vi "Broadcast Origin.vi"(8 "error in (no error)":errorcluster, 11 "Yaml Model in":refnum<class "Yaml Model.lvclass">) -> (0 "error out":errorcluster, 3 "Yaml Model out":refnum<class "Yaml Model.lvclass">)   [LabVIEW 2020, in "Yaml Model.lvlib" / "Yaml Model.lvclass"]
uses:
  Yaml Model.lvclass
  Yaml Model Messages/Abstract Origin Msg/Abstract Origin Msg.lvclass
  C:/Program Files/National Instruments/LabVIEW 2020/vi.lib/ActorFrameworkObserver/Data Message/Data Message.lvclass
  Yaml Model.lvclass/Yaml Model.ctl
  <vilib>/ActorFrameworkObserver/Actor Register/Actor Register.lvclass
panel:
  # "NOTICE -- YOU MUST LEAVE THIS NOTICE IN PLACE.\n\nCopyright (c) 2017, LIANG LIU Shawn.Liu.cn@gmail.com\nAll rights reserved.\n\nRedistribution and use in source and binary forms, with or without modification, are permitted provided that the following conditions are met:\n-Redistributions of source code must retain the above copyright notice, this list of conditions and the following disclaimer.\n-Redistributions in binary form must reproduce the above copyright notice, this list of conditions and the following disclaimer in the documentation and/or other materials provided with the distribution.\n-Neither the name of the eLp nor the names of its contributors may be used to endorse or promote products derived from this software without specific prior written permission.\n\nTHIS SOFTWARE IS PROVIDED BY THE COPYRIGHT HOLDERS AND CONTRIBUTORS \"AS IS\" AND ANY EXPRESS OR IMPLIED WARRANTIES, INCLUDING, BUT NOT LIMITED TO, THE IMPLIED WARRANTIES OF MERCHANTABILITY AND FITNESS FOR A PARTICULAR PURPOSE ARE DISCLAIMED. IN NO EVENT SHALL THE COPYRIGHT HOLDER OR CONTRIBUTORS BE LIABLE FOR ANY DIRECT, INDIRECT, INCIDENTAL, SPECIAL, EXEMPLARY, OR CONSEQUENTIAL DAMAGES (INCLUDING, BUT NOT LIMITED TO, PROCUREMENT OF SUBSTITUTE GOODS OR SERVICES; LOSS OF USE, DATA, OR PROFITS; OR BUSINESS INTERRUPTION) HOWEVER CAUSED AND ON ANY THEORY OF LIABILITY, WHETHER IN CONTRACT, STRICT LIABILITY, OR TORT (INCLUDING NEGLIGENCE OR OTHERWISE) ARISING IN ANY WAY OUT OF THE USE OF THIS SOFTWARE, EVEN IF ADVISED OF THE POSSIBILITY OF SUCH DAMAGE."
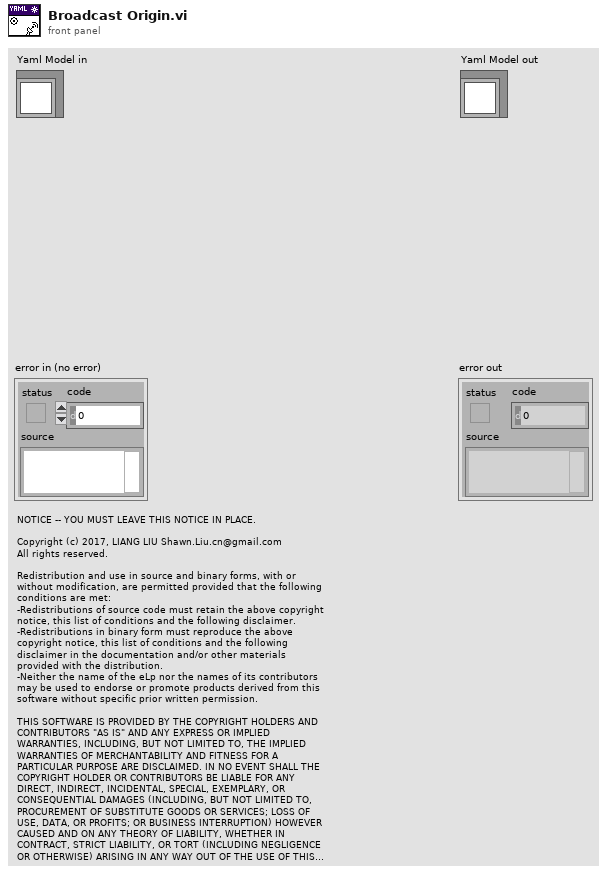
[diagram p1: front panel]
types:
  T1 = cluster{"Image":string, "Resolution":dbl, "Origin":cluster{"X":dbl, "Y":dbl, "R":dbl}, "Occupied Thresh":dbl, "Free Thresh":dbl, "Negate":bool}
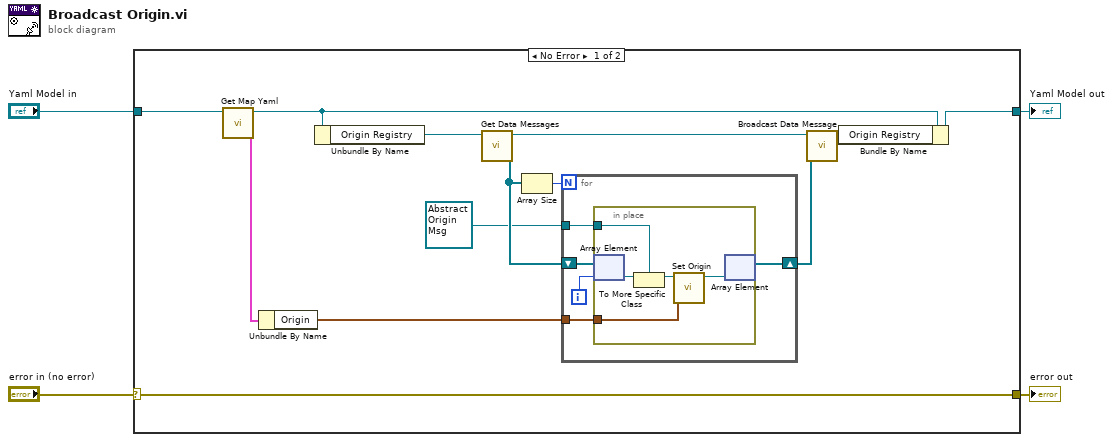
[diagram p0: block diagram]
diagram:
  n1 = case "Error Case" shown="No Error" "error in (no error)" {
    selector: "error in (no error)" -> [w8 w29]
    tunnel: "Yaml Model in" -> [w17 w28]
    tunnel: [w16 w28] -> w3
    tunnel: [w8 w29] -> w2
    frame No Error {
      n2 = call "Get Map Yaml.vi"("Yaml Model in"=w17) -> ("Map Yaml"=w6:T1, "Yaml Model out"=w7:refnum<class "Yaml Model.lvclass">)  [unwired: 9 in]
      n3 = Unbundle By Name(w6) -> ("Origin"=w5:cluster{"X":dbl, "Y":dbl, "R":dbl})
      n4 = Unbundle By Name(w7) -> ("Origin Registry"=w15:refnum<class "Actor Register.lvclass">)
      n5 = call-dynamic "Get Data Messages.vi"("Actor Register in"=w15) -> ("Data Messages"=w12:refnum<class "Data Message.lvclass">[], "Actor Register out"=w14:refnum<class "Actor Register.lvclass">)  [unwired: 9 in]
      n6 = Array Size(array=w12) -> (size(s)=w10:i32)
      n7 = for {
        N: w10 -> [_]
        shift-right: [w20] -> w9
        shift-left: w12 -> [w22]
        tunnel: refnum<class "Abstract Origin Msg.lvclass"> refnum ("Yaml Model.lvlib:Abstract Origin Msg.lvclass") -> [w21]
        tunnel: w5 -> [w18]
        i -> [w19]
        n8 = in-place {
          in-place-border: w21 -> [w26]
          in-place-border: w18 -> [w23]
          n9 = in-place-array #1(w22, w19) -> (w27:refnum<class "Data Message.lvclass">)
          n10 = To More Specific Class(target class=w26, reference=w27) -> (specific class reference=w25:refnum<class "Abstract Origin Msg.lvclass">)  [unwired: 1 in, 1 out]
          n11 = call "Set Origin.vi"("Origin"=w23, "Abstract Origin Msg in"=w25) -> ("Abstract Origin Msg out"=w24:refnum<class "Abstract Origin Msg.lvclass">)  [unwired: 9 in]
          n12 = in-place-array #1(w24) -> (w20:refnum<class "Data Message.lvclass">[])  [unwired: 1 out]
        }
      }
      n13 = call <vilib>:"Broadcast Data Message.vi"("Data Messages"=w9, "Actor Register in"=w14) -> ("Actor Register out"=w13:refnum<class "Actor Register.lvclass">)  [unwired: 8 in, 1 out]
      n14 = Bundle By Name(cluster=w7, "Origin Registry"=w13) -> (w16:refnum<class "Yaml Model.lvclass">)
    }
    frame Error {
    }
  }
  "error out" <- w2
  "Yaml Model out" <- w3
